vi "Get Request Type.vi"(8 "error in (no error)":errorcluster, 11 "GetInputList in":refnum<class "GetInputList.lvclass">) -> (0 "error out":errorcluster, 2 "Request Type":string, 3 "GetInputList out":refnum<class "GetInputList.lvclass">)   [LabVIEW 2020, in "obs-websocket.lvlib" / "GetInputList.lvclass"]
uses:
  GetInputList.lvclass
  GetInputList.lvclass/GetInputList.ctl
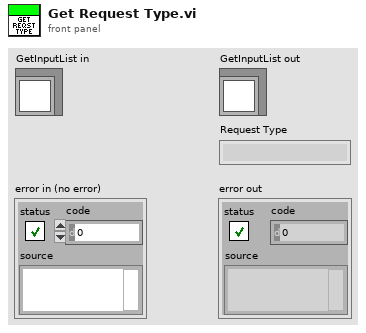
[diagram p1: front panel]
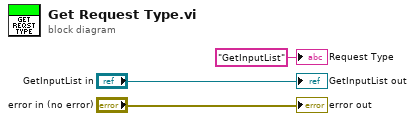
[diagram p0: block diagram]
diagram:
  "error out" <- "error in (no error)"
  "GetInputList out" <- "GetInputList in"
  "Request Type" <- "GetInputList" ("Request Type")
